vi "getGroupDof.vi"(8 "error in (no error)":errorcluster, 9 "Input DOF":dbl[](array[numeric]), 10 "DOF Group":T1, 11 "ZTAAC in":refnum<class "ZTAAC.lvclass">) -> (0 "error out":errorcluster, 2 "DOF":dbl[](array[numeric]), 3 "ZTAAC out":refnum<class "ZTAAC.lvclass">)   [LabVIEW 2016, in "OfcFunc.lvlib" / "ZTAAC.lvclass"]
doc: "Get the degree of freedom (DOF) of specific group:\n1. M2 hexapod position (dz in um, dx in um, dy in um, rx in arcsec, ry in arcsec).\n2. Cam hexapod position (dz in um, dx in um, dy in um, rx in arcsec, ry in arcsec).\n3. M1M3 20 bending mode in um.\n4. M2 20 bending mode in um.\n\n* If there is no input DOF, the output will be the aggregated DOF (state - state0)."
uses:
  ZTAAC.lvclass
  StrictDef/DofGroup.ctl
  ZTAAC.lvclass/ZTAAC.ctl
  OptCtrl/OptCtrl.lvclass
  OptStateEsti/OptStateEsti.lvclass
  OfcFunc.lvlib
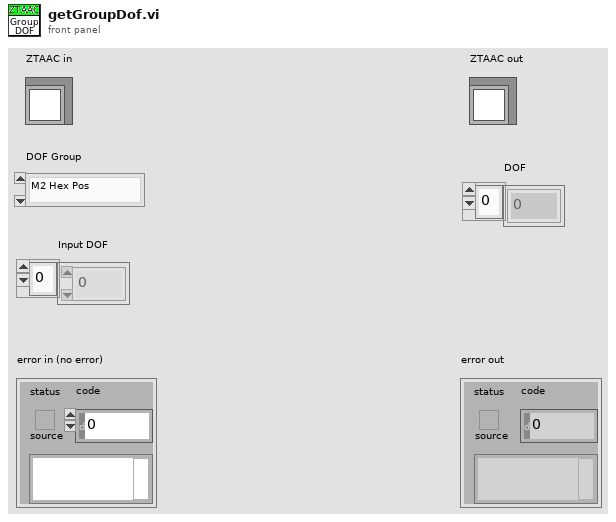
[diagram p1: front panel]
types:
  T1 = typedef "OfcFunc.lvlib/DofGroup.ctl" = enum16{"M2 Hex Pos", "Cam Hex Pos", "M1M3 Bend", "M2 Bend"}
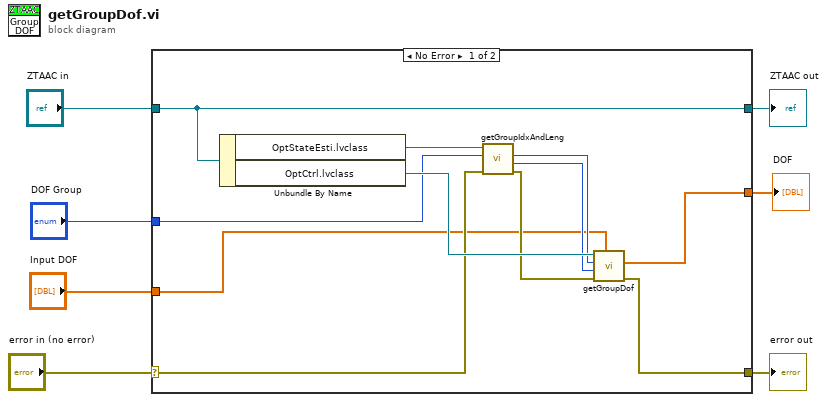
[diagram p0: block diagram]
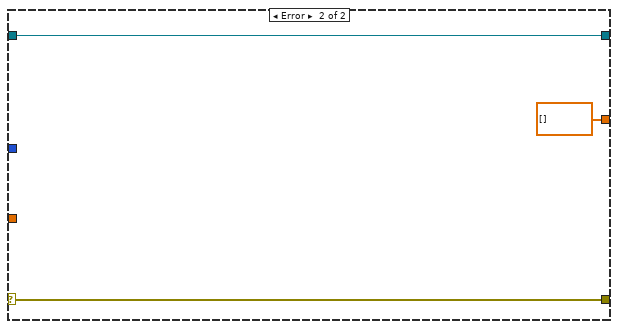
[diagram p2: hidden frame]
diagram:
  n1 = case shown="No Error" "error in (no error)" {
    selector: "error in (no error)" -> [w12 w21]
    tunnel: [w15 w21] -> w6
    tunnel: [w18 w20] -> w4
    tunnel: "ZTAAC in" -> [w18 w20]
    tunnel: "DOF Group" -> [w13 _]
    tunnel: [w16 dbl[] [] ("DOF")] -> w2
    tunnel: "Input DOF" -> [w8 _]
    frame No Error {
      n2 = Unbundle By Name(w18) -> ("OptStateEsti.lvclass"=w14:refnum<class "OptStateEsti.lvclass">, "OptCtrl.lvclass"=w17:refnum<class "OptCtrl.lvclass">)
      n3 = call "getGroupIdxAndLeng.vi"("error in (no error)"=w12, "DOF Group"=w13, "OptStateEsti in"=w14) -> ("error out"=w11:errorcluster, "Group Length"=w9:i32, "Start Index"=w10:i32)  [unwired: 5 in, 1 out]
      n4 = call "getGroupDof.vi"("Input DOF"=w8, "error in (no error)"=w11, "Group Length"=w9, "Start Index"=w10, "OptCtrl in"=w17) -> ("error out"=w15:errorcluster, "DOF"=w16:dbl[])  [unwired: 4 in, 1 out]
    }
    frame Error {
    }
  }
  "error out" <- w6
  "ZTAAC out" <- w4
  "DOF" <- w2
